vi "Handle Error.vi"(8 "error in (no error)":errorcluster, 11 "Command Actor in":refnum<class "Command Actor.lvclass">) -> (0 "error out":errorcluster, 2 "stop actor?":bool=TRUE, 3 "Command Actor out":refnum<class "Command Actor.lvclass">)   [LabVIEW 2014, in "Robot Actor Framework.lvlib" / "Command Actor.lvlib" / "Command Actor.lvclass"]
doc: "(<B>Filename</B>: Actor Framework.lvlib:Actor.lvclass:Handle Error.vi)\n\nDefines how the actor handles an error that occurred while processing a message. By default, this method does nothing except stop the actor."
uses:
  Command Actor.lvclass
  <vilib>/ni/Actors/State Actor/State Actor/State Actor.lvclass
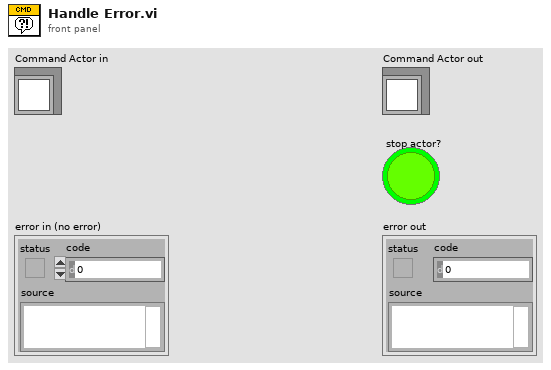
[diagram p1: front panel]
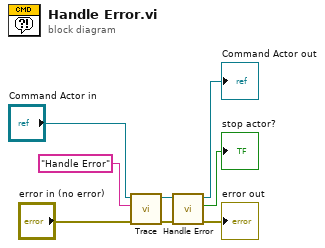
[diagram p0: block diagram]
diagram:
  n1 = call-dynamic "Trace.vi"("error in (no error)"="error in (no error)", "Command Action"="Handle Error", "Command Actor in"="Command Actor in") -> ("error out"=w3:errorcluster, "Command Actor out"=w1:refnum<class "Command Actor.lvclass">)  [unwired: 7 in]
  n2 = call-parent "Handle Error.vi"("error in (no error)"=w3, "Actor in"=w1) -> ("error out"=→"error out":errorcluster, "stop actor?"=→"stop actor?":bool, "Actor out"=→"Command Actor out":refnum<class "Command Actor.lvclass">)  [unwired: 7 in]
